vi "FP behavior P-Wall.vi"(1 "Behavior\nVelocity":dbl=20.0, 2 "Activate?":bool=TRUE, 3 "IR Sensors":T1(array[cluster])) -> (0 "P-Wall Array":dbl[](array[numeric]))   [LabVIEW 2014]
doc: "This vi creates a array based upon the value of the PBow IR sensor reading."
uses:
  <vilib>/addons/control/pid/pid.llb/PID (DBL).vi
  <vilib>/addons/control/pid/NI_PID_pid.lvlib
panel:
  in  "setpoint":dbl=40.0 format="%#_13g"
  out "steer":dbl format="%.2f"
  out "Sensor \nbeing used":string
  out "Waveform Graph":cluster{dbl, dbl, dbl[]}(graph)
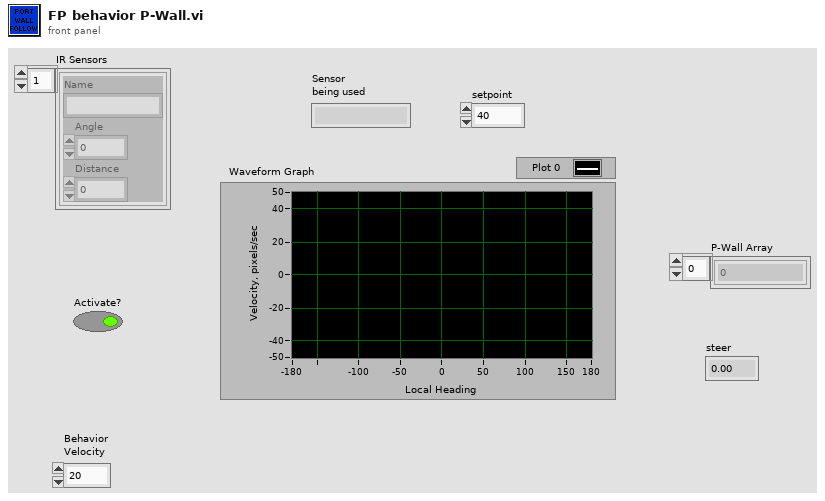
[diagram p1: front panel]
types:
  T1 = cluster{"Name":string, "Angle":dbl, "Distance":dbl}[]
  T2 = cluster{"proportional gain (Kc)":dbl, "integral time (Ti, min)":dbl, "derivative time (Td, min)":dbl}
  T3 = cluster{"Name":string, "Angle":dbl, "Distance":dbl}
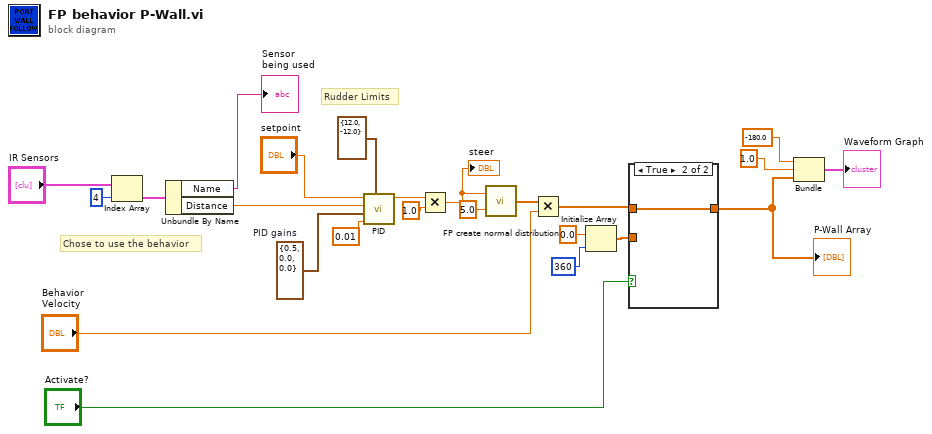
[diagram p0: block diagram]
diagram:
  w8 = T2 {"proportional gain (Kc)"=0.5, "integral time (Ti, min)"=0.0, "derivative time (Td, min)"=0.0}  # PID gains
  # "Rudder Limits"
  # "Chose to use the behavior"
  n1 = Index Array(array="IR Sensors", index=4) -> (element=w15:T3)
  n2 = Unbundle By Name(w15) -> ("Name"=→"Sensor \nbeing used":string, "Distance"=w7:dbl)
  n3 = call-poly <vilib>:"PID.vi"("output range"=cluster{"output high":dbl, "output low":dbl} {"output high"=12.0, "output low"=-12.0}, "dt (s)"=0.01, "PID gains"=w8, "process variable"=w7, "setpoint"="setpoint") -> ("output"=w12:dbl)  [unwired: 5 in, 1 out]
  n4 = Multiply(x=w12, y=1.0) -> (x*y=w6:dbl)
  "steer" <- w6
  n5 = call "FP create normal distribution.vi"("std (Normal)"=5.0, "mean"=w6) -> ("ACT array"=w5:dbl[])
  n6 = Multiply(x=w5, y="Behavior\nVelocity") -> (x*y=w4:dbl[])
  n7 = Initialize Array(0.0 ("element"), 360 ("dimension size")) -> (w18:dbl[])
  n8 = case shown="True" "Activate?" {
    tunnel: w18 -> [w25 _]
    tunnel: w4 -> [_ w26]
    tunnel: [w25 w26] -> w17
    frame False {
    }
    frame True {
    }
  }
  "P-Wall Array" <- w17
  n9 = Bundle(-180.0, 1.0, w17) -> (→"Waveform Graph":cluster{dbl, dbl, dbl[]})  [unwired: 1 in]
